vi "Logging_using_sqlite.vi"() -> ()   [LabVIEW 2016]
uses:
  <vilib>/drjdpowell/SQLite Library/SQL Statement/SQL Statement.lvclass/SQL Statement.ctl
  <vilib>/drjdpowell/SQLite Library/SQL Connection/Open (path).vi
  <vilib>/drjdpowell/SQLite Library/SQL Statement/Bind Timestamp.vi
  <vilib>/drjdpowell/SQLite Library/SQL Statement/Bind Text.vi
  <vilib>/drjdpowell/SQLite Library/SQL Statement/Bind Real.vi
  <vilib>/drjdpowell/SQLite Library/SQL Statement/Bind Integer.vi
  <vilib>/NI/Current Value Table/DataTypes/U16_Read.vi
  <vilib>/NI/Current Value Table/DataTypes/Boolean_Read.vi
  <vilib>/drjdpowell/SQLite Library/SQL Statement/Bind Timestamp (Real).vi
  <vilib>/drjdpowell/SQLite Library/SQL Connection/Open (string).vi
  <vilib>/drjdpowell/SQLite Library/SQL Statement/Step.vi
  <vilib>/drjdpowell/SQLite Library/SQL Statement/Bind Blob.vi
  <vilib>/NI/Current Value Table/Type to Enum.vi
  <vilib>/NI/Current Value Table/DataTypes/U16_Type To Enum.vi
  <vilib>/NI/Current Value Table/DataTypes/Boolean_Type To Enum.vi
  <vilib>/Utility/file.llb/Read Delimited Spreadsheet (string).vi
  <vilib>/AdvancedString/Path To Command Line String.vi
  <vilib>/drjdpowell/SQLite Library/SQL Connection/Execute SQL (No results).vi
  <vilib>/drjdpowell/SQLite Library/SQL Statement/Error Message.vi
  <vilib>/NI/Current Value Table/FGVs/CVT Globals.vi
  <vilib>/NI/Current Value Table/FGVs/Tag Memory.vi
  <vilib>/NI/Current Value Table/Memory Block.vi
  <vilib>/NI/Current Value Table/DataTypes/U16_Memory Block.vi
  <vilib>/NI/Current Value Table/DataTypes/Boolean_Memory Block.vi
  <vilib>/drjdpowell/SQLite Library/SQL Connection/Connection.lvclass
  <vilib>/drjdpowell/SQLite Library/SQL Statement/SQL Statement.lvclass
  <vilib>/NI/Current Value Table/Current Value Table.lvlib
  <vilib>/drjdpowell/SQLite Library/SQLite.lvlib
panel:
  in  "Time Stamp":timestamp
  in  "Array":string[](array[string])
  in  "I64":i64
  in  "Numeric2":dbl
  in  "Knob2":dbl(knob) scale=0.0..10.0
  in  "Numeric1":dbl
  in  "String (update while typing)":string
  in  "String":string
  in  "Knob1":dbl(knob) scale=0.0..10.0
  in  "Slide2":dbl(slide) scale=0.0..10.0
  in  "Slide1":dbl(slide) scale=0.0..10.0
  in  "stop":bool
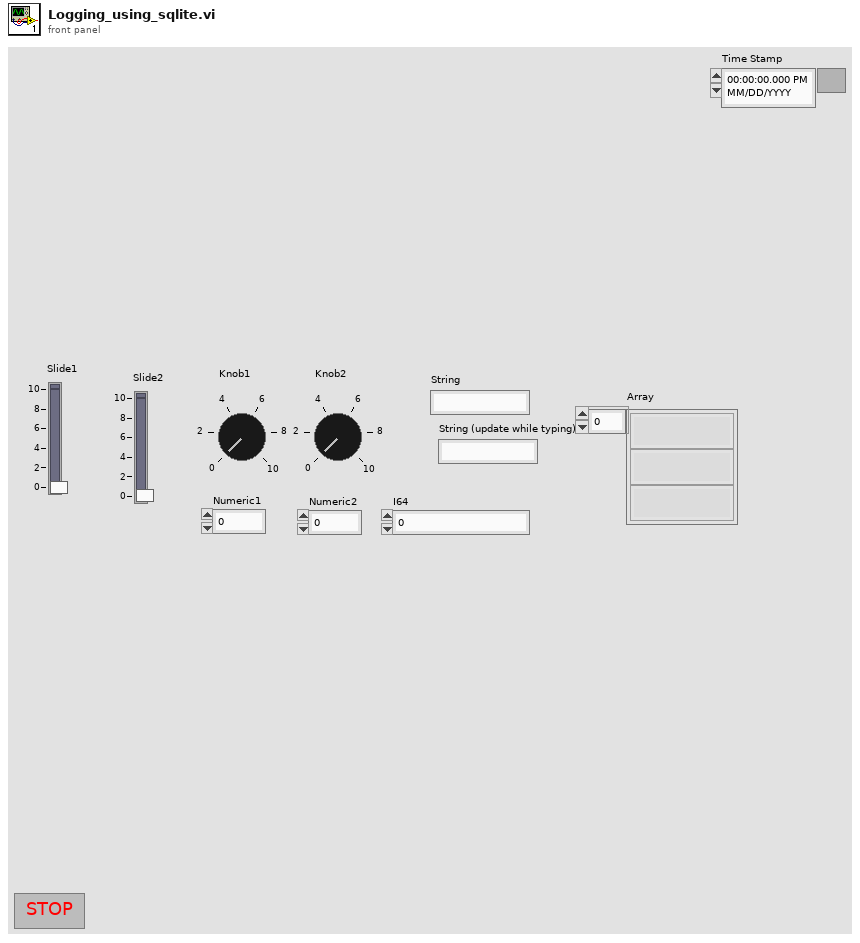
[diagram p1: front panel]
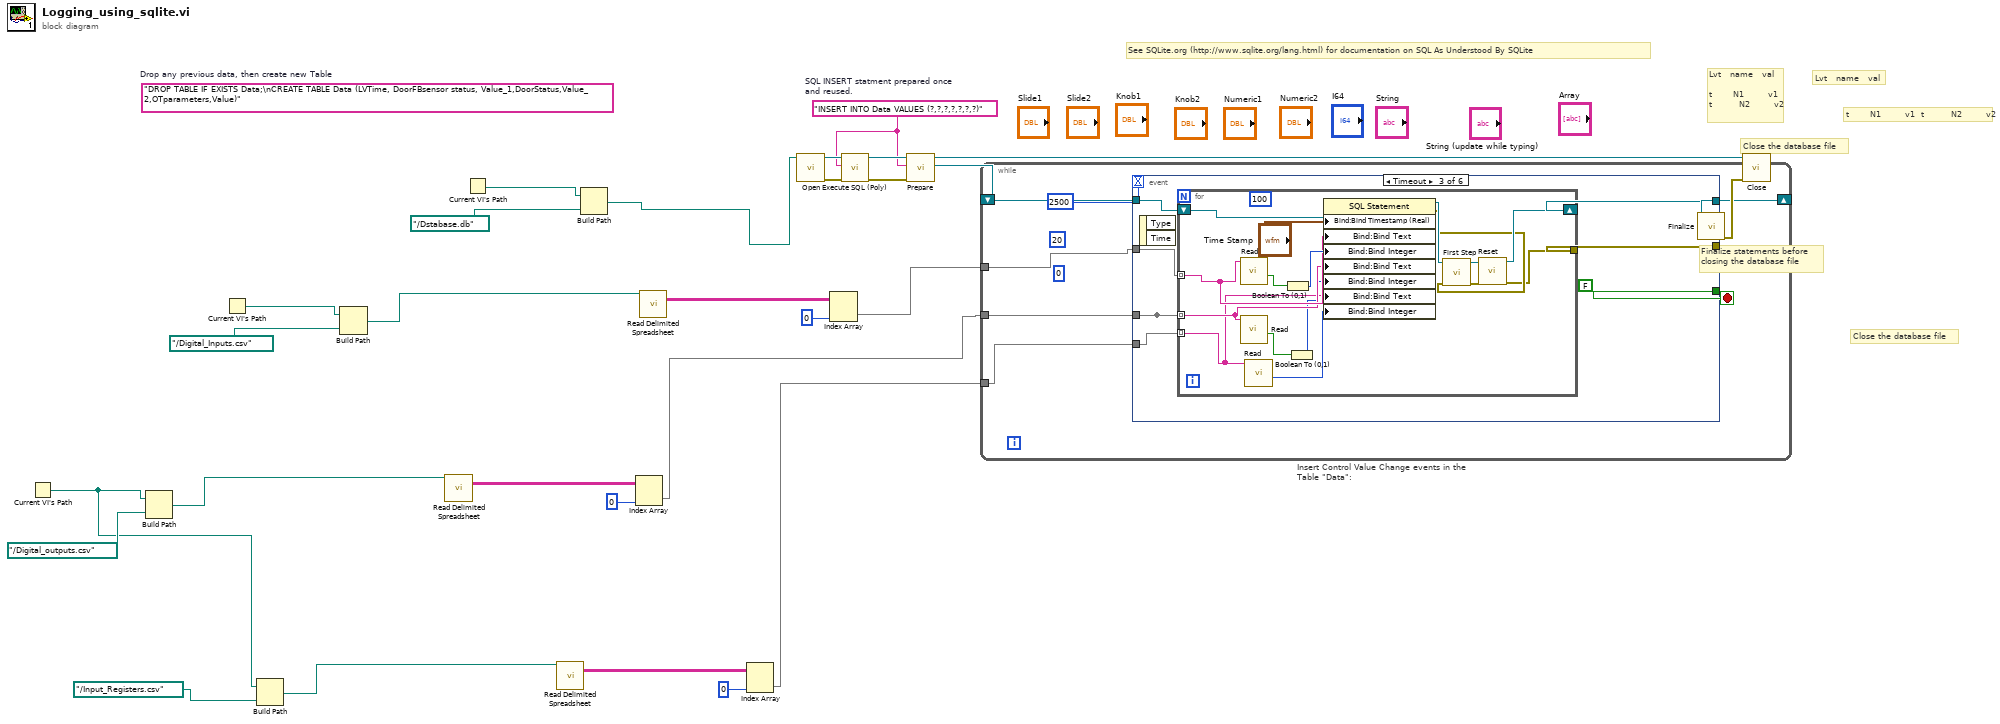
[diagram p0: block diagram]
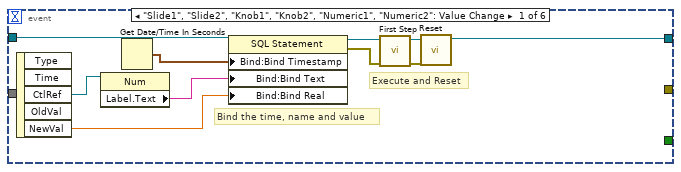
[diagram p2: hidden frame]
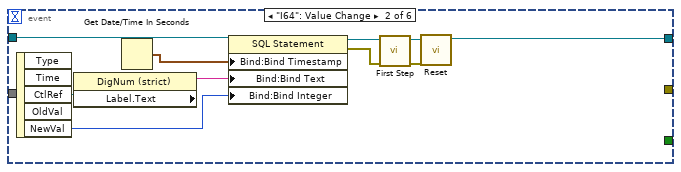
[diagram p3: hidden frame]
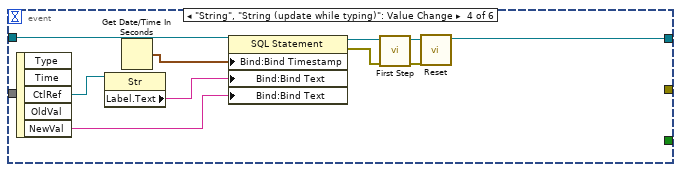
[diagram p4: hidden frame]
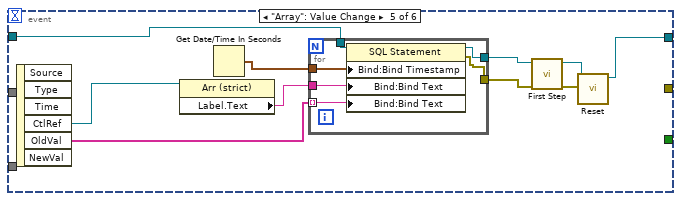
[diagram p5: hidden frame]
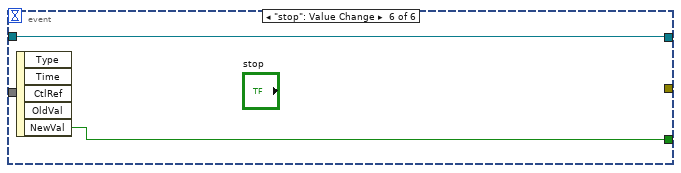
[diagram p6: hidden frame]
diagram:
  w1 = "INSERT INTO Data VALUES (?,?,?,?,?,?,?)"  # SQL INSERT statment prepared once and reused.
  (unwired) "DROP TABLE IF EXISTS Data;\nCREATE TABLE Data (LVTime, DoorFBsensor status, Value_1,DoorStatus,Value_2,OTparameters,Value)"  # Drop any previous data, then create new Table
  # "t       N1        v1  t         N2        v2"
  # "Lvt   name   val"
  # "Lvt   name   val\n\nt       N1        v1\nt         N2        v2"
  # "Finalize statements before\nclosing the database file"
  # "Close the database file"
  # "Close the database file"
  # "See SQLite.org (http://www.sqlite.org/lang.html) for documentation on SQL As Understood By SQLite"
  n1 = Current VI's Path() -> (path=w2:path)
  n2 = Build Path(base path=w2, name or relative path=path "../Digital_outputs.csv") -> (appended path=w11:path)
  n3 = Current VI's Path() -> (path=w20:path)
  n4 = Build Path(base path=w2, name or relative path=path "../Input_Registers.csv") -> (appended path=w7:path)
  n5 = Build Path(base path=w20, name or relative path=path "../Digital_Inputs.csv") -> (appended path=w18:path)
  n6 = call-poly <vilib>:"Read Delimited Spreadsheet.vi"("file path (dialog if empty)"=w11) -> ("all rows"=w10:string[][])  [unwired: 9 in, 5 out]
  n7 = Current VI's Path() -> (path=w15:path)
  n8 = call-poly <vilib>:"Read Delimited Spreadsheet.vi"("file path (dialog if empty)"=w7) -> ("all rows"=w6:string[][])  [unwired: 9 in, 5 out]
  n9 = Build Path(base path=w15, name or relative path=path "../Dstabase.db") -> (appended path=w13:path)
  n10 = Index Array "Index Array"(array=w10, index (col)=0 ("disabled index (col)")) -> (element=w9:string[])  [unwired: 1 in]
  n11 = call-poly <vilib>:"Read Delimited Spreadsheet.vi"("file path (dialog if empty)"=w18) -> ("all rows"=w17:string[][])  [unwired: 9 in, 5 out]
  n12 = Index Array "Index Array"(array=w6, index (col)=0 ("disabled index (col)")) -> (element=w5:string[])  [unwired: 1 in]
  n13 = call-poly <vilib>:"Open.vi"("db file"=w13) -> ("error out"=w28:errorcluster, "SQLite Connection"=w29:refnum<class "Connection.lvclass">)  [unwired: 9 in]
  n14 = Index Array "Index Array"(array=w17, index (col)=0 ("disabled index (col)")) -> (element=w16:string[])  [unwired: 1 in]
  n15 = call-poly <vilib>:"Execute SQL (Poly).vi"("error in (no error)"=w28, "SQL"=w1, "SQLite Connection in"=w29) -> ("error out"=w23:errorcluster, "SQLite Connection"=w27:refnum<class "Connection.lvclass">)  [unwired: 7 in]
  n16 = call <vilib>:"Prepare.vi"("error in (no error)"=w23, "SQL"=w1, "SQLite Connection in"=w27) -> ("SQL Statement"=w26:refnum<class "SQL Statement.lvclass">, "SQLite Connection"=w25:refnum<class "Connection.lvclass">)  [unwired: 4 in, 3 out]
  n17 = while "Insert Control Value Change events in the Table \"Data\":" {
    shift-right: [w34] -> w22
    shift-left: w26 -> [w35]
    tunnel: w16 -> [w32]
    tunnel: w9 -> [w31]
    tunnel: w5 -> [w30]
    stop <- w36 stop-if-true
    (unwired) u16 20 ("quantity")
    (unwired) u16 0 ("starting address")
    n18 = event shown="[2] Timeout" {
      selector: _ -> [_ _ _ _ _ _]
      dyn-events: _ -> [_ _ _ _ _ _]
      timeout: 2500 ("Numeric") -> [_ _ _ _ _ _]
      tunnel: [_ _ _ _ _ w105] -> w36
      tunnel: w35 -> [w46 w56 w62 w88 w95 w106]
      tunnel: [w41 w51 w61 w83 w90 w106] -> w34
      tunnel: [_ _ w60 _ _ _] -> _
      tunnel: w32 -> [_ _ w59 _ _ _]
      tunnel: [_ _ w58 _ _ _] -> _
      tunnel: w31 -> [_ _ w58 _ _ _]
      tunnel: w30 -> [_ _ w57 _ _ _]
      event "Slide1", "Slide2", "Knob1", "Knob2", "Numeric1", "Numeric2": Value Change {
        # "Bind the time, name and value"
        # "Execute and Reset"
        n19 = event-data() -> ("CtlRef"=w40:refnum<vi>, "NewVal"=w37:dbl)  [unwired: 1 in, 3 out]
        n20 = property class="Num"(reference=w40) -> ("Label.Text"=w39:string)  [unwired: 1 in, 2 out]
        n21 = Get Date/Time In Seconds() -> (seconds since 1Jan1904=w38:timestamp)
        n22 = property class="SQL Statement"(reference=w46, "Bind:Bind Timestamp"=w38, "Bind:Bind Text"=w39, "Bind:Bind Real"=w37) -> (reference out=w44:refnum<class "SQL Statement.lvclass">, error out=w45:errorcluster)  [unwired: 1 in]
        n23 = call <vilib>:"First Step.vi"("error in (no error)"=w45, "SQL Statement in"=w44) -> ("error out"=w43:errorcluster, "SQL Statement"=w42:refnum<class "SQL Statement.lvclass">)  [unwired: 7 in, 1 out]
        n24 = call <vilib>:"Reset.vi"("error in (no error)"=w43, "SQL Statement in"=w42) -> ("SQL Statement"=w41:refnum<class "SQL Statement.lvclass">)  [unwired: 8 in, 1 out]
      }
      event "I64": Value Change {
        n25 = event-data() -> ("CtlRef"=w50:refnum<vi>, "NewVal"=w47:i64)  [unwired: 1 in, 3 out]
        n26 = property class="DigNum (strict)"(reference=w50) -> ("Label.Text"=w49:string)  [unwired: 1 in, 2 out]
        n27 = Get Date/Time In Seconds() -> (seconds since 1Jan1904=w48:timestamp)
        n28 = property class="SQL Statement"(reference=w56, "Bind:Bind Timestamp"=w48, "Bind:Bind Text"=w49, "Bind:Bind Integer"=w47) -> (reference out=w54:refnum<class "SQL Statement.lvclass">, error out=w55:errorcluster)  [unwired: 1 in]
        n29 = call <vilib>:"First Step.vi"("error in (no error)"=w55, "SQL Statement in"=w54) -> ("error out"=w53:errorcluster, "SQL Statement"=w52:refnum<class "SQL Statement.lvclass">)  [unwired: 7 in, 1 out]
        n30 = call <vilib>:"Reset.vi"("error in (no error)"=w53, "SQL Statement in"=w52) -> ("SQL Statement"=w51:refnum<class "SQL Statement.lvclass">)  [unwired: 8 in, 1 out]
      }
      event Timeout {
        (unwired) FALSE
        n31 = event-data() -> ()  [unwired: 1 in, 2 out]
        n32 = for {
          shift-right: [w73] -> w61
          shift-left: w62 -> [w78]
          tunnel: [w71] -> w60
          tunnel: w59 -> [w69] mode=indexing
          tunnel: w58 -> [w68] mode=indexing
          tunnel: w57 -> [w65] mode=indexing
          (unwired) 100
          n33 = call-poly <vilib>:"Read.vi"("Tag Name"=w69) -> ("Value"=w70:bool)  [unwired: 9 in, 1 out]
          n34 = call-poly <vilib>:"Read.vi"("Tag Name"=w68) -> ("Value"=w67:bool)  [unwired: 9 in, 1 out]
          n35 = call-poly <vilib>:"Read.vi"("Tag Name"=w65) -> ("Value"=w64:u16)  [unwired: 9 in, 1 out]
          n36 = Boolean To (0,1)(Boolean=w70) -> (0, 1=w77:i16)
          n37 = Boolean To (0,1)(Boolean=w67) -> (0, 1=w66:i16)
          n38 = property class="SQL Statement"(reference=w78, "Bind:Bind Timestamp (Real)"="Time Stamp", "Bind:Bind Text"=w69, "Bind:Bind Integer"=w77, "Bind:Bind Text"=w68, "Bind:Bind Integer"=w66, "Bind:Bind Text"=w65, "Bind:Bind Integer"=w64) -> (reference out=w74:refnum<class "SQL Statement.lvclass">, error out=w72:errorcluster)  [unwired: 1 in]
          n39 = call <vilib>:"First Step.vi"("error in (no error)"=w72, "SQL Statement in"=w74) -> ("error out"=w75:errorcluster, "SQL Statement"=w76:refnum<class "SQL Statement.lvclass">)  [unwired: 7 in, 1 out]
          n40 = call <vilib>:"Reset.vi"("error in (no error)"=w75, "SQL Statement in"=w76) -> ("error out"=w71:errorcluster, "SQL Statement"=w73:refnum<class "SQL Statement.lvclass">)  [unwired: 8 in]
        }
      }
      event "String", "String (update while typing)": Value Change {
        n41 = event-data() -> ("CtlRef"=w82:refnum<vi>, "NewVal"=w79:string)  [unwired: 1 in, 3 out]
        n42 = property class="Str"(reference=w82) -> ("Label.Text"=w81:string)  [unwired: 1 in, 2 out]
        n43 = Get Date/Time In Seconds() -> (seconds since 1Jan1904=w80:timestamp)
        n44 = property class="SQL Statement"(reference=w88, "Bind:Bind Timestamp"=w80, "Bind:Bind Text"=w81, "Bind:Bind Text"=w79) -> (reference out=w86:refnum<class "SQL Statement.lvclass">, error out=w87:errorcluster)  [unwired: 1 in]
        n45 = call <vilib>:"First Step.vi"("error in (no error)"=w87, "SQL Statement in"=w86) -> ("error out"=w85:errorcluster, "SQL Statement"=w84:refnum<class "SQL Statement.lvclass">)  [unwired: 7 in, 1 out]
        n46 = call <vilib>:"Reset.vi"("error in (no error)"=w85, "SQL Statement in"=w84) -> ("SQL Statement"=w83:refnum<class "SQL Statement.lvclass">)  [unwired: 8 in, 1 out]
      }
      event "Array": Value Change {
        n47 = event-data() -> ("CtlRef"=w89:refnum<vi>, "OldVal"=w96:string[])  [unwired: 1 in, 4 out]
        n48 = property class="Arr (strict)"(reference=w89) -> ("Label.Text"=w98:string)  [unwired: 1 in, 2 out]
        n49 = Get Date/Time In Seconds() -> (seconds since 1Jan1904=w97:timestamp)
        n50 = for {
          tunnel: w98 -> [w104]
          tunnel: w97 -> [w103]
          tunnel: w96 -> [w102] mode=indexing
          tunnel: w95 -> [w101]
          tunnel: [w100] -> w92
          tunnel: [w99] -> w91
          n51 = property class="SQL Statement"(reference=w101, "Bind:Bind Timestamp"=w103, "Bind:Bind Text"=w104, "Bind:Bind Text"=w102) -> (reference out=w100:refnum<class "SQL Statement.lvclass">, error out=w99:errorcluster)  [unwired: 1 in]
        }
        n52 = call <vilib>:"First Step.vi"("error in (no error)"=w91, "SQL Statement in"=w92) -> ("error out"=w94:errorcluster, "SQL Statement"=w93:refnum<class "SQL Statement.lvclass">)  [unwired: 7 in, 1 out]
        n53 = call <vilib>:"Reset.vi"("error in (no error)"=w94, "SQL Statement in"=w93) -> ("SQL Statement"=w90:refnum<class "SQL Statement.lvclass">)  [unwired: 8 in, 1 out]
      }
      event "stop": Value Change {
        n54 = event-data() -> ("NewVal"=w105:bool)  [unwired: 1 in, 4 out]
      }
    }
  }
  n55 = call <vilib>:"Finalize.vi"("SQL Statement in"=w22) -> ("error out"=w24:errorcluster)  [unwired: 10 in]
  n56 = call-dynamic "Close.vi"("error in (no error)"=w24, "SQLite Connection in"=w25) -> ()  [unwired: 9 in, 1 out]
